vi "short_cmd_read.vi"(5 "COM":bool, 7 "VISA name":refnum<visa-resource-name>, 8 "data":u8[](array[numeric]), 9 "dwLen":u16, 10 "dwAddr":u16, 11 "cmd_short_header_t":T1) -> (2 "return":i32, 3 "data out":u8[](array[numeric]))   [LabVIEW 2016]
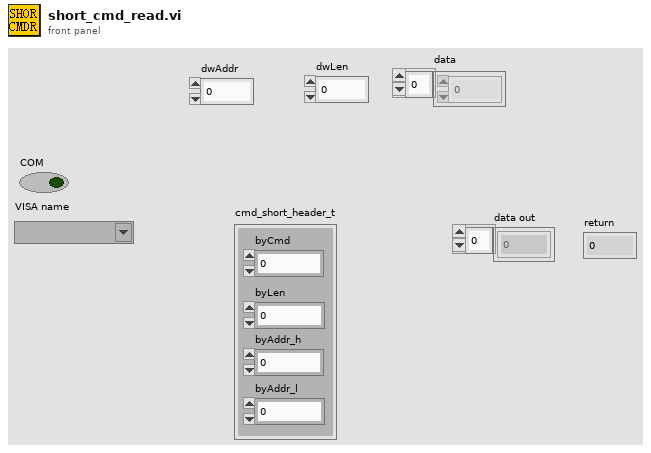
[diagram p1: front panel]
types:
  T1 = cluster{"byCmd":u8, "byLen":u8, "byAddr_h":u8, "byAddr_l":u8}
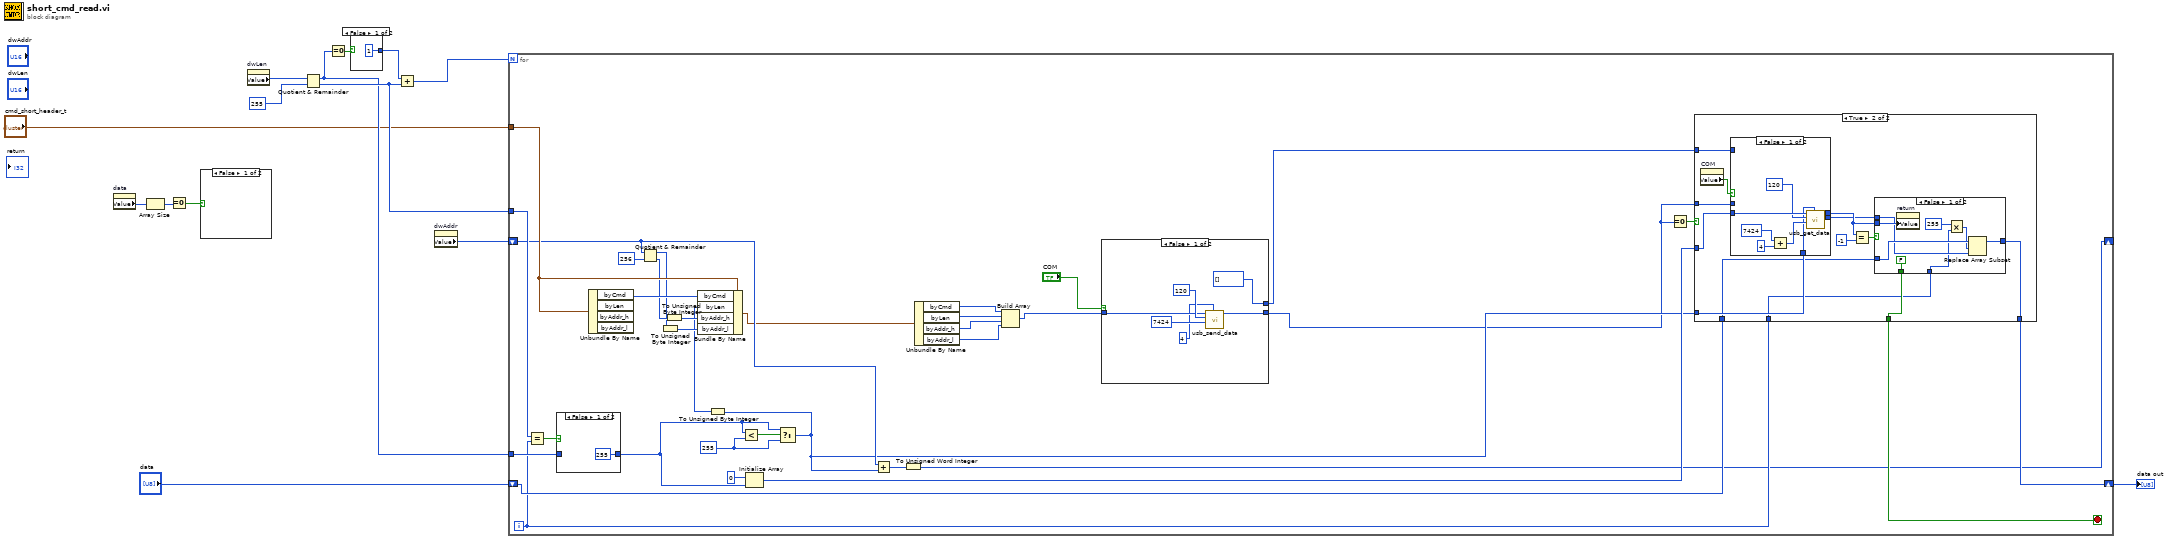
[diagram p0: block diagram]
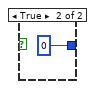
[diagram p2: hidden frame]
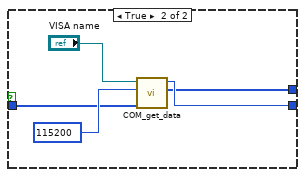
[diagram p3: hidden frame]
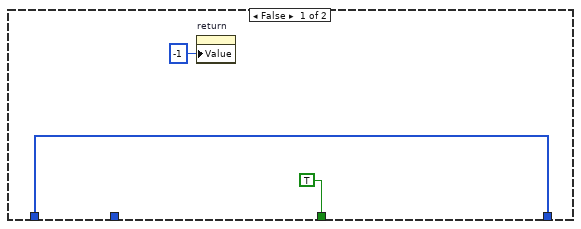
[diagram p5: hidden frame]
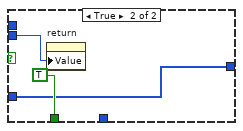
[diagram p7: hidden frame]
diagram:
  n1 = property on="data" class="Arr (strict)"() -> ("Value"=w14:u8[])  [unwired: 2 in, 2 out]
  n2 = Array Size(array=w14) -> (size(s)=w12:i32)
  n3 = Equal To 0?(x=w12) -> (x = 0?=w13:bool)
  n4 = case shown="False" w13 {
    frame False {
    }
    frame True {
    }
  }
  n5 = property on="dwLen" class="DigNum (strict)"() -> ("Value"=w11:u16)  [unwired: 2 in, 2 out]
  n6 = Quotient & Remainder(x=w11, y=u16 255) -> (x-y*floor(x/y)=w5:u16, floor(x/y)=w6:u16)
  n7 = Equal To 0?(x=w5) -> (x = 0?=w9:bool)
  n8 = case shown="False" w9 {
    tunnel: [u32 1 u32 0] -> w8
    frame False {
    }
    frame True {
    }
  }
  n9 = Add(x=w8, y=w6) -> (x+y=w7:u32)
  n10 = property on="dwAddr" class="DigNum (strict)"() -> ("Value"=w3:u16)  [unwired: 2 in, 2 out]
  n11 = for {
    N: w7 -> [_]
    tunnel: w6 -> [w45]
    tunnel: w5 -> [w44]
    shift-right: [w39] -> w2
    shift-left: "data" -> [w40]
    tunnel: "cmd_short_header_t" -> [w37]
    shift-right: [w34] -> _
    shift-left: w3 -> [w33]
    i -> [w38]
    stop <- w47 stop-if-true
    w49 = u16 255 ("f")
    n12 = Equal?(x=w45, y=w38) -> (x = y?=w46:bool)
    n13 = case shown="False" w46 {
      tunnel: w44 -> [_ w63]
      tunnel: [u16 255 w63] -> w42
      frame False {
      }
      frame True {
      }
    }
    n14 = Unbundle By Name(w37) -> ("byCmd"=w36:u8)  [unwired: 3 out]
    n15 = Quotient & Remainder(x=w33, y=u16 256) -> (x-y*floor(x/y)=w30:u16, floor(x/y)=w31:u16)
    n16 = To Unsigned Byte Integer(number=w30) -> (unsigned 8bit integer=w29:u8)
    n17 = To Unsigned Byte Integer(number=w31) -> (unsigned 8bit integer=w28:u8)
    n18 = Less?(x=w42, y=w49) -> (x < y?=w50:bool)
    n19 = Initialize Array(u8 0 ("element"), w42) -> (w41:u8[])
    n20 = Select(t=w42, s=w50, f=w49) -> (s? t:f=w27:u16)
    n21 = To Unsigned Byte Integer(number=w27) -> (unsigned 8bit integer=w26:u8)
    n22 = Bundle By Name(cluster=w37, "byCmd"=w36, "byLen"=w26, "byAddr_h"=w28, "byAddr_l"=w29) -> (w25:T1)
    n23 = Add(x=w33, y=w27) -> (x+y=w35:u16)
    n24 = To Unsigned Word Integer(number=w35) -> (unsigned 16bit integer=w34:u16)
    n25 = Unbundle By Name(w25) -> ("byCmd"=w24:u8, "byLen"=w23:u8, "byAddr_h"=w22:u8, "byAddr_l"=w21:u8)
    n26 = Build Array(w24, w23, w22, w21) -> (w20:u8[])
    n27 = case shown="False" "COM" {
      tunnel: w20 -> [w54 w59]
      tunnel: [w53 w58] -> w17
      tunnel: [u8[] [] ("data out") w57] -> w18
      frame False {
        n28 = call "usb_send_data.vi"("byVdCmdHeaderLen"=u16 4, "I2C_VD_BUFFER_RW"=u16 7424, "I2C_SLAVE_ID"=u8 120, "data"=w54) -> ("return"=w53:i32)  [unwired: 6 in, 1 out]
      }
      frame True {
        n29 = call "COM_get_data.vi"("data"=w59, "baud rate (9600)"=u32 115200, "VISA name"="VISA name") -> ("data out"=w57:u8[], "return"=w58:i32)  [unwired: 7 in]
      }
    }
    n30 = Equal To 0?(x=w17) -> (x = 0?=w48:bool)
    n31 = case shown="True" w48 {
      tunnel: [TRUE w75] -> w47
      tunnel: w41 -> [_ w79]
      tunnel: w27 -> [_ w78]
      tunnel: w40 -> [w64 w73]
      tunnel: [w64 w70] -> w39
      tunnel: w38 -> [_ w71]
      tunnel: w18 -> [_ w68]
      tunnel: w17 -> [_ w67]
      frame False {
        n32 = property on="return" class="DigNum (strict)"("Value"=-1 ("return")) -> ()  [unwired: 2 in, 2 out]
      }
      frame True {
        n33 = property on="COM" class="Bool (strict)"() -> ("Value"=w69:bool)  [unwired: 2 in, 2 out]
        n34 = case shown="False" w69 {
          tunnel: w79 -> [w87 _]
          tunnel: w78 -> [w80 _]
          tunnel: [w82 w89] -> w74
          tunnel: [w81 w88] -> w72
          tunnel: w68 -> [_ w88]
          tunnel: w67 -> [_ w89]
          frame False {
            n35 = Add(x=u16 7424 ("I2C_VD_BUFFER_RW"), y=u16 4) -> (x+y=w83:u16)
            n36 = call "usb_get_data.vi"("byVdCmdHeaderLen"=w80, "I2C_VD_BUFFER_RW"=w83, "I2C_SLAVE_ID"=u8 120, "data"=w87) -> ("data out"=w81:u8[], "return"=w82:i32)  [unwired: 5 in, 1 out]
          }
          frame True {
          }
        }
        n37 = Equal?(x=w74, y=-1) -> (x = y?=w77:bool)
        n38 = case shown="False" w77 {
          tunnel: [FALSE TRUE] -> w75
          tunnel: w74 -> [w96 w99]
          tunnel: w73 -> [w95 w98]
          tunnel: w72 -> [w94 _]
          tunnel: w71 -> [w92 _]
          tunnel: [w90 w98] -> w70
          frame False {
            n39 = property on="return" class="DigNum (strict)"("Value"=w96) -> ()  [unwired: 2 in, 2 out]
            n40 = Multiply(x=255, y=w92) -> (x*y=w91:i32)
            n41 = Replace Array Subset(array=w95, new element=w94, index=w91) -> (w90:u8[])
          }
          frame True {
            n42 = property on="return" class="DigNum (strict)"("Value"=w99) -> ()  [unwired: 2 in, 2 out]
          }
        }
      }
    }
  }
  "data out" <- w2
